vi "8 PATTEN.vi"() -> ()   [LabVIEW 2017]
panel:
  in  "Numeric":u8
  out "E":bool
  out "F":bool
  out "B":bool
  out "C":bool
  out "D":bool
  out "G":bool
  out "A":bool
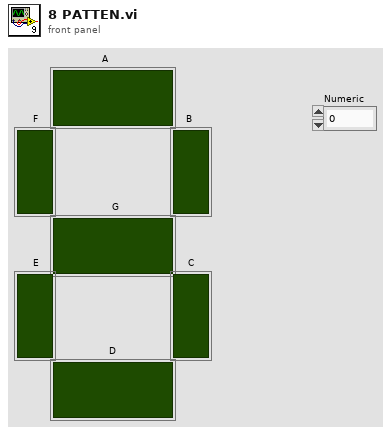
[diagram p1: front panel]
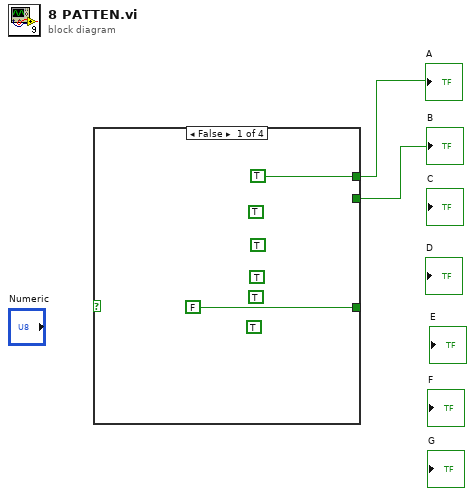
[diagram p0: block diagram]
diagram:
  n1 = case shown="\"0\"" {
    selector: _ -> [_ _ _ _]
    tunnel: [TRUE _ _ _] -> w2
    tunnel: [FALSE _ _ _] -> _
    tunnel: [_ _ _ _] -> w1
    frame False {
      (unwired) TRUE
      (unwired) TRUE
      (unwired) TRUE
      (unwired) TRUE
      (unwired) TRUE
    }
    frame True {
    }
    frame True {
    }
    frame True {
    }
  }
  "A" <- w2
  "B" <- w1
